vi "Configure I2C.vi"(0 "Data Source":T2={"Data Source (0:Channel1)"=0, "Data Threshold (1.2V)"=1.2} {"Data Source (0:Channel1)" items=["Channel 1", "Channel 2", "Channel 3", "Channel 4"]}, 5 "Clock Source":T1={"Clock Source (1:Channel2) "=1, "Clock Threshold (1.2V)"=1.2} {"Clock Source (1:Channel2)" items=["Channel 1", "Channel 2", "Channel 3", "Channel 4"]}, 7 "Trigger On (0:Start)":u16(ring) items=["Start", "Stop", "Repeated Start", "Missing ack", "Address", "Data", "Address And Data"], 9 "Data Direction (0:Either)":u16(ring) items=["Either", "Read", "Write"], 11 "Addressing Mode (0:7 Bit)":u16(ring) items=["7 Bit", "10 Bit"]) -> (8 "Output String":string)   [LabVIEW 2011, in "Tektronix 7000 Series.lvlib"]
doc: "Configures the common settings for the I2C trigger."
uses:
  Tektronix 7000 Series.lvlib
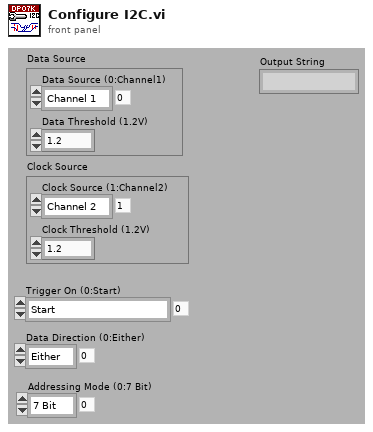
[diagram p1: front panel]
types:
  T1 = cluster{"Clock Source (1:Channel2) ":u16, "Clock Threshold (1.2V)":dbl}
  T2 = cluster{"Data Source (0:Channel1)":u16, "Data Threshold (1.2V)":dbl}
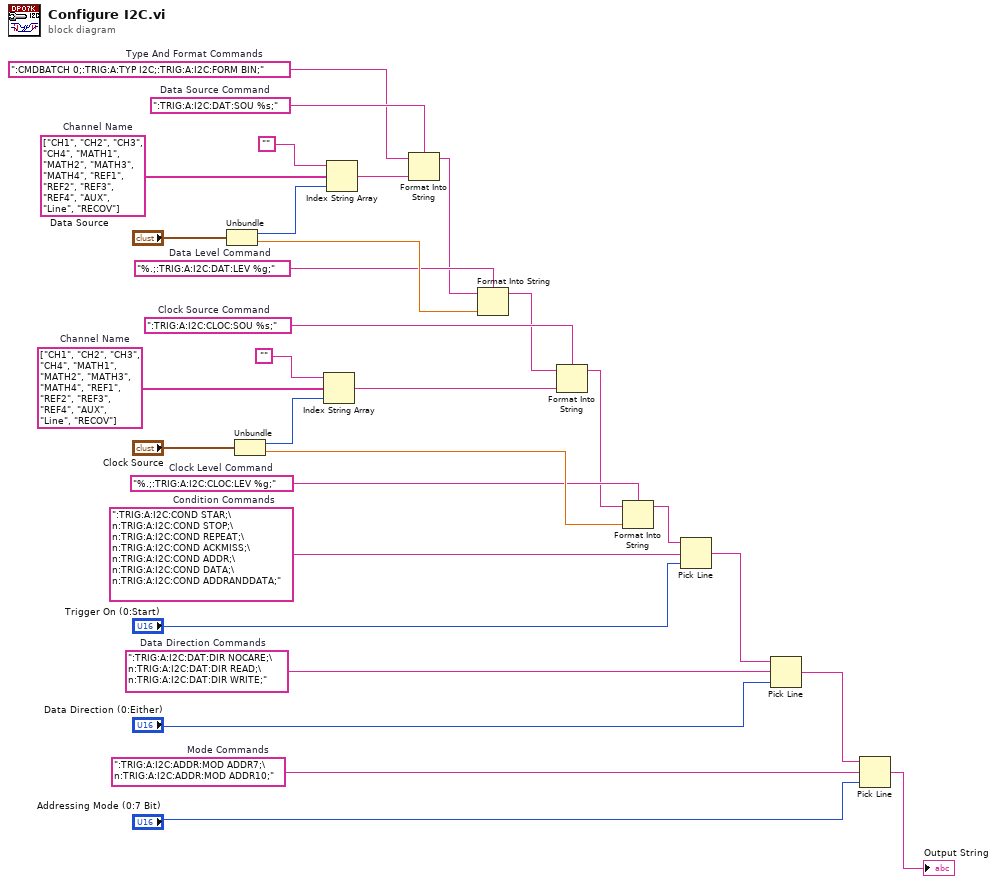
[diagram p0: block diagram]
diagram:
  w29 = ":TRIG:A:I2C:ADDR:MOD ADDR7;\n:TRIG:A:I2C:ADDR:MOD ADDR10;"  # Mode Commands
  w27 = ":TRIG:A:I2C:DAT:DIR NOCARE;\n:TRIG:A:I2C:DAT:DIR READ;\n:TRIG:A:I2C:DAT:DIR WRITE;"  # Data Direction Commands
  w25 = ":TRIG:A:I2C:COND STAR;\n:TRIG:A:I2C:COND STOP;\n:TRIG:A:I2C:COND REPEAT;\n:TRIG:A:I2C:COND ACKMISS;\n:TRIG:A:I2C:COND ADDR;\n:TRIG:A:I2C:COND DATA;\n:TRIG:A:I2C:COND ADDRANDDATA;"  # Condition Commands
  w22 = "%.;:TRIG:A:I2C:CLOC:LEV %g;"  # Clock Level Command
  w20 = ":TRIG:A:I2C:CLOC:SOU %s;"  # Clock Source Command
  w16 = string[] ["CH1", "CH2", "CH3", "CH4", "MATH1", "MATH2", "MATH3", "MATH4", "REF1", "REF2", "REF3", "REF4", "AUX", "Line", "RECOV"]  # Channel Name
  w13 = "%.;:TRIG:A:I2C:DAT:LEV %g;"  # Data Level Command
  w10 = ":CMDBATCH 0;:TRIG:A:TYP I2C;:TRIG:A:I2C:FORM BIN;"  # Type And Format Commands
  w11 = ":TRIG:A:I2C:DAT:SOU %s;"  # Data Source Command
  w7 = string[] ["CH1", "CH2", "CH3", "CH4", "MATH1", "MATH2", "MATH3", "MATH4", "REF1", "REF2", "REF3", "REF4", "AUX", "Line", "RECOV"]  # Channel Name
  n1 = Unbundle("Data Source") -> ("Data Source (0:Channel1)"=w8:u16, "Data Threshold (1.2V)"=w14:dbl)
  n2 = Unbundle("Clock Source") -> ("Clock Source (1:Channel2)"=w17:u16, "Clock Threshold (1.2V)"=w23:dbl)
  n3 = Index String Array(1:w17, 2:w16, 3:"" ("Empty String Constant")) -> (0:w19:string)
  n4 = Index String Array(1:w8, 2:w7, 3:"" ("Empty String Constant")) -> (0:w9:string)
  n5 = Format Into String(format string=w11, initial string=w10, w9) -> (resulting string=w12:string)  [unwired: 1 in, 1 out]
  n6 = Format Into String(format string=w13, initial string=w12, w14) -> (resulting string=w18:string)  [unwired: 1 in, 1 out]
  n7 = Format Into String(format string=w20, initial string=w18, w19) -> (resulting string=w21:string)  [unwired: 1 in, 1 out]
  n8 = Format Into String(format string=w22, initial string=w21, w23) -> (resulting string=w24:string)  [unwired: 1 in, 1 out]
  n9 = Pick Line(string ("")=w24, multi-line string=w25, line index="Trigger On (0:Start)") -> (output string=w26:string)
  n10 = Pick Line(string ("")=w26, multi-line string=w27, line index="Data Direction (0:Either)") -> (output string=w28:string)
  n11 = Pick Line(string ("")=w28, multi-line string=w29, line index="Addressing Mode (0:7 Bit)") -> (output string=→"Output String":string)
